vi "onProcessStop.vi"(8 "error in (no error)":errorcluster, 11 "SMO":refnum<class "SMO.lvclass">) -> (0 "error out":errorcluster, 3 "SMO out":refnum<class "SMO.lvclass">)   [LabVIEW 2021, in "smo.lvlib" / "SMO.lvclass"]
uses:
  SMO.lvclass
  SMO.lvclass/SMO.ctl
panel:
  # "For instructions on how to use the JKI State Machine Objects, examples and video tutorials, visit:\nhttp://jki.net/state-machine-objects/\n\nJKI State Machine Objects™\nhttp://jki.net/state-machine-objects/\nCopyright (C) 2005-2015, JKI <info@jki.net>\nALL RIGHTS RESERVED"
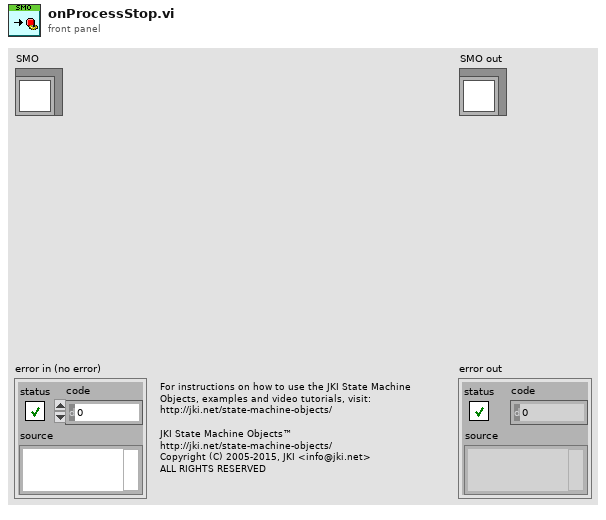
[diagram p1: front panel]
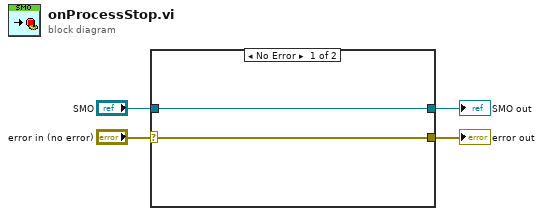
[diagram p0: block diagram]
diagram:
  n1 = case shown="No Error" "error in (no error)" {
    selector: "error in (no error)" -> [w5 w8]
    tunnel: [w5 w8] -> w3
    tunnel: [w6 w7] -> w1
    tunnel: "SMO" -> [w6 w7]
    frame No Error {
    }
    frame Error {
    }
  }
  "error out" <- w3
  "SMO out" <- w1
